vi "MGCC_combs.vi"(9 "v":dbl[](array[numeric]), 10 "m":i32) -> (1 "P":T1)   [LabVIEW 2016]
uses:
  <vilib>/Analysis/Matrix/Datatypes/RealMatrix.ctl
  <vilib>/Analysis/Matrix/Numeric/Conversions/Array To Matrix - RA.vi
  <vilib>/Analysis/Matrix/Numeric/Conversions/Array To Matrix - RA2.vi
  <vilib>/Analysis/Matrix/NI_Matrix.lvlib
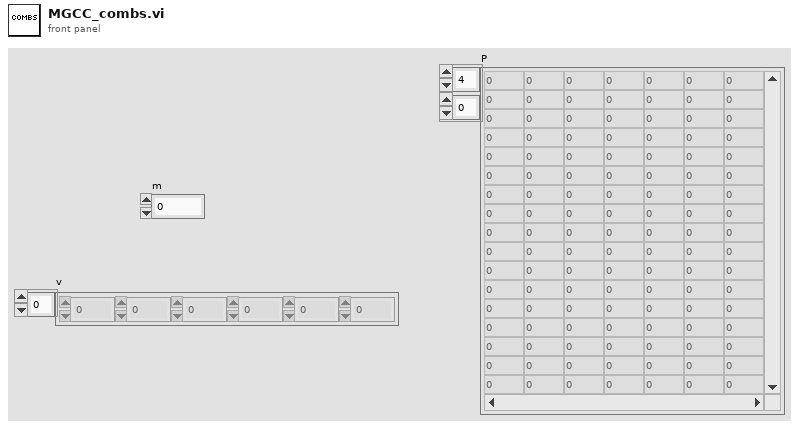
[diagram p1: front panel]
types:
  T1 = typedef "NI_Matrix.lvlib/RealMatrix.ctl" = dbl[][]
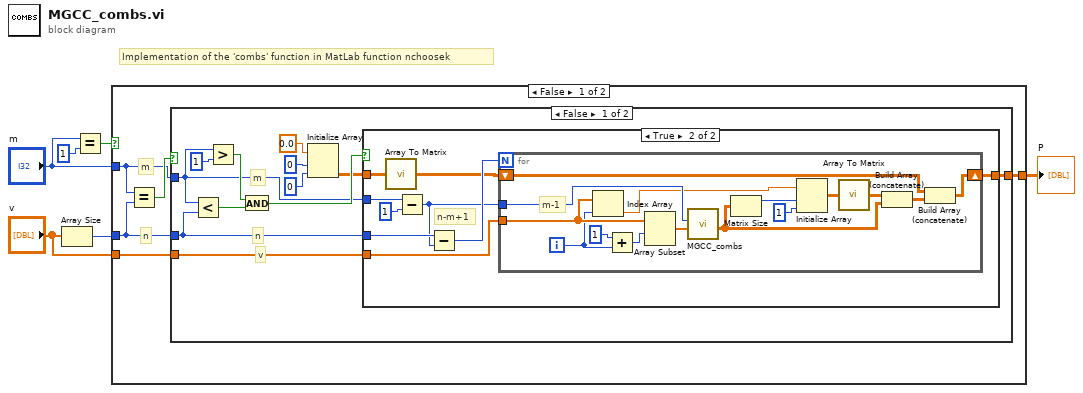
[diagram p0: block diagram]
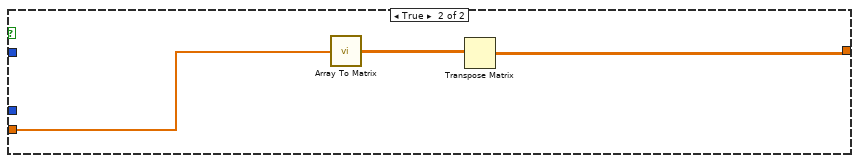
[diagram p3: hidden frame]
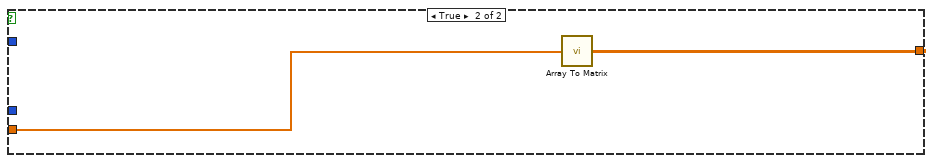
[diagram p4: hidden frame]
diagram:
  # "Implementation of the 'combs' function in MatLab function nchoosek"
  n1 = Array Size(array="v") -> (size(s)=w4:i32)
  n2 = Equal?(x="m", y=1) -> (x = y?=w6:bool)
  n3 = case shown="False" w6 {
    tunnel: [w10 w52] -> w2
    tunnel: "m" -> [w8 _]
    tunnel: w4 -> [w9 _]
    tunnel: "v" -> [w7 w53]
    frame False {
      # "n"
      # "m"
      n4 = Equal?(x=w8, y=w9) -> (x = y?=w11:bool)
      n5 = case shown="False" w11 {
        tunnel: [w12 w49] -> w10
        tunnel: w9 -> [w16 _]
        tunnel: w8 -> [w15 _]
        tunnel: w7 -> [w14 w51]
        frame False {
          # "v"
          # "n"
          # "m"
          n6 = Less?(x=w15, y=w16) -> (x < y?=w19:bool)
          n7 = Greater?(x=w15, y=1) -> (0:w18:bool)
          n8 = And(x=w18, y=w19) -> (x .and. y?=w17:bool)
          n9 = Initialize Array(0.0 ("element"), 0 ("dimension size"), 0 ("dimension size")) -> (w13:dbl[][])
          n10 = case shown="True" w17 {
            tunnel: w16 -> [_ w32]
            tunnel: w15 -> [_ w30]
            tunnel: w14 -> [_ w28]
            tunnel: w13 -> [w24 w27]
            tunnel: [w24 w25] -> w12
            frame False {
            }
            frame True {
              # "n-m+1"
              n11 = call-poly <vilib>:"Array To Matrix.vi"("Real 2D Array"=w27) -> ("Real Matrix"=w26:T1)
              n12 = Subtract(x=w30, y=1) -> (x-y=w29:i32)
              n13 = Subtract(x=w32, y=w29) -> (x-y=w31:i32)
              n14 = for {
                N: w31 -> [_]
                tunnel: w29 -> [w48]
                tunnel: w28 -> [w44]
                shift-right: [w37] -> w25
                shift-left: w26 -> [w39]
                i -> [w34]
                # "m-1"
                n15 = Index Array(array=w44, index=w34) -> (element=w43:dbl)
                n16 = Add(x=1, y=w34) -> (x+y=w35:i32)
                n17 = Array Subset(array=w44, index=w35) -> (w47:dbl[])  [unwired: 1 in]
                n18 = call "MGCC_combs.vi"("v"=w47, "m"=w48) -> ("P"=w40:T1)  [unwired: 9 in]
                n19 = Matrix Size(0:w40) -> (1:w45:i32)  [unwired: 1 out]
                n20 = Initialize Array(w43, w45, 1 ("dimension size")) -> (w42:dbl[][])
                n21 = call-poly <vilib>:"Array To Matrix.vi"("Real 2D Array"=w42) -> ("Real Matrix"=w41:T1)
                n22 = Build Array (concatenate)(w41, w40) -> (w38:T1)
                n23 = Build Array (concatenate)(w39, w38) -> (w37:T1)
              }
            }
          }
        }
        frame True {
          n24 = call-poly <vilib>:"Array To Matrix.vi"("Real 1D Array"=w51) -> ("Real Matrix (Column Vector)"=w50:T1)
          n25 = Transpose Matrix(1:w50) -> (0:w49:T1)
        }
      }
    }
    frame True {
      n26 = call-poly <vilib>:"Array To Matrix.vi"("Real 1D Array"=w53) -> ("Real Matrix (Column Vector)"=w52:T1)
    }
  }
  "P" <- w2
